vi "kaisser.vi"(0 "Banda Transicion (normalizada)":dbl=0.2, 1 "delta (rizado)":dbl=0.01) -> (2 "A (db)":dbl=20.0, 3 "Beta":dbl, 4 "N+1":i32=9)   [LabVIEW 2020]
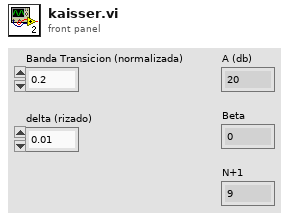
[diagram p1: front panel]
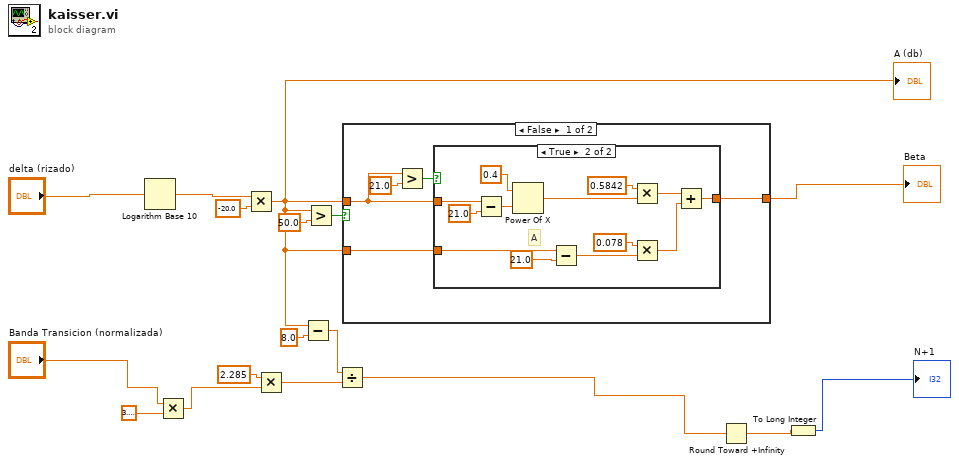
[diagram p0: block diagram]
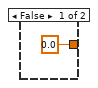
[diagram p2: hidden frame]
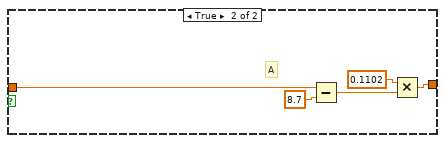
[diagram p3: hidden frame]
diagram:
  n1 = Logarithm Base 10(1:"delta (rizado)") -> (0:w8:dbl)
  n2 = Multiply(x="Banda Transicion (normalizada)", y=3.141592653589793) -> (x*y=w3:dbl)
  n3 = Multiply(x=w8, y=-20.0) -> (x*y=w17:dbl)
  "A (db)" <- w17
  n4 = Multiply(x=2.285, y=w3) -> (x*y=w12:dbl)
  n5 = Subtract(x=w17, y=8.0) -> (x-y=w10:dbl)
  n6 = Greater?(x=w17, y=50.0) -> (0:w14:bool)
  n7 = Divide(x=w10, y=w12) -> (x/y=w16:dbl)
  n8 = case shown="False" w14 {
    tunnel: w17 -> [w19 w38]
    tunnel: [w20 w37] -> w15
    tunnel: w17 -> [w18 _]
    frame False {
      n9 = Greater?(x=w19, y=21.0) -> (0:w21:bool)
      n10 = case shown="True" w21 {
        tunnel: [0.0 ("y") w26] -> w20
        tunnel: w19 -> [_ w25]
        tunnel: w18 -> [_ w24]
        frame False {
        }
        frame True {
          # "A"
          n11 = Subtract(x=w25, y=21.0) -> (x-y=w31:dbl)
          n12 = Power Of X(1:w31, 2:0.4 ("y")) -> (0:w29:dbl)
          n13 = Subtract(x=w24, y=21.0) -> (x-y=w34:dbl)
          n14 = Multiply(x=0.5842, y=w29) -> (x*y=w28:dbl)
          n15 = Multiply(x=0.078, y=w34) -> (x*y=w27:dbl)
          n16 = Add(x=w28, y=w27) -> (x+y=w26:dbl)
        }
      }
    }
    frame True {
      # "A"
      n17 = Subtract(x=w38, y=8.7) -> (x-y=w41:dbl)
      n18 = Multiply(x=0.1102, y=w41) -> (x*y=w37:dbl)
    }
  }
  "Beta" <- w15
  n19 = Round Toward +Infinity(x=w16) -> (ceil(x): smallest int >= x=w2:dbl)
  n20 = To Long Integer(number=w2) -> (32bit integer=→"N+1":i32)
